vi "Log_subVI.vi"(6 "Data B":fxp<+,16,3>[](array[numeric]), 7 "Data A":fxp<+,16,3>[](array[numeric]), 8 "error in (no error)":errorcluster, 9 "Path":path, 10 "Samples to Read":dbl, 11 "Amplitude (V)":dbl) -> (0 "error out":errorcluster, 3 "Echo":dbl[][](graph))   [LabVIEW 2017]
doc: "Logs data from two separate channels and writes them to a single file on disk."
uses:
  <vilib>/Utility/file.llb/Write Delimited Spreadsheet (string).vi
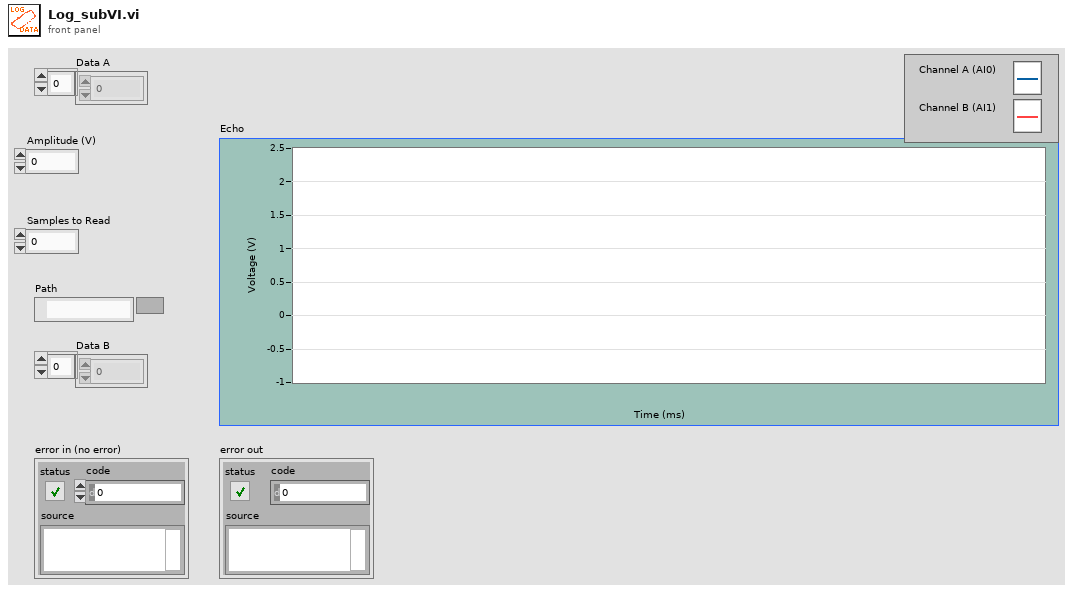
[diagram p1: front panel]
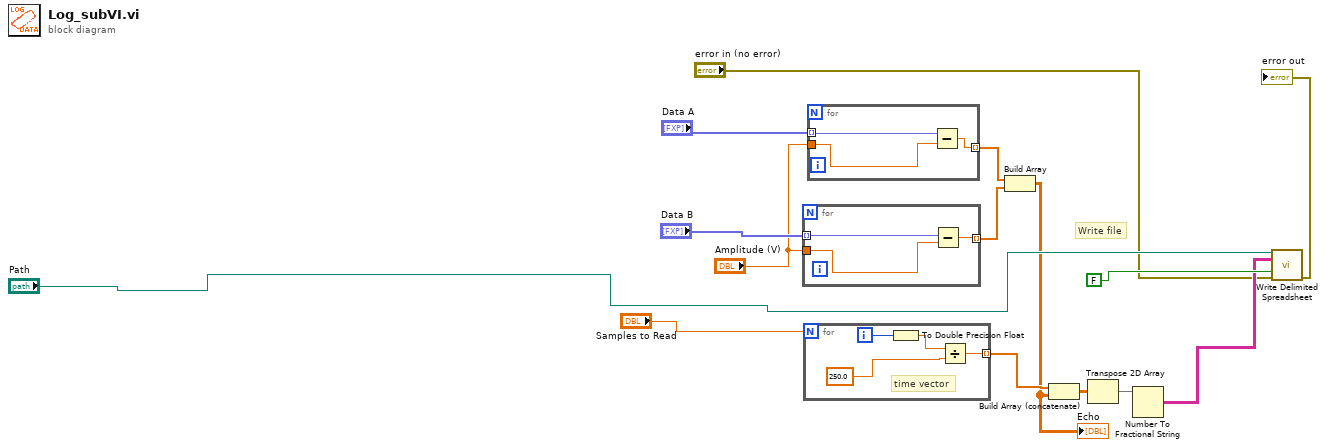
[diagram p0: block diagram]
diagram:
  # "Write file"
  n1 = for {
    tunnel: "Data B" -> [w18] mode=indexing
    tunnel: [w17] -> w12 mode=indexing
    tunnel: "Amplitude (V)" -> [w16]
    n2 = Subtract(x=w18, y=w16) -> (x-y=w17:dbl)
  }
  n3 = for {
    N: "Samples to Read" -> [_]
    tunnel: [w20] -> w10 mode=indexing
    i -> [w22]
    # "time vector"
    n4 = To Double Precision Float(number=w22) -> (double precision float=w21:dbl)
    n5 = Divide(x=w21, y=250.0) -> (x/y=w20:dbl)
  }
  n6 = for {
    tunnel: "Data A" -> [w25] mode=indexing
    tunnel: [w24] -> w11 mode=indexing
    tunnel: "Amplitude (V)" -> [w23]
    n7 = Subtract(x=w25, y=w23) -> (x-y=w24:dbl)
  }
  n8 = Build Array(w11, w12) -> (w7:dbl[][])
  "Echo" <- w7
  n9 = Build Array (concatenate)(w10, w7) -> (w8:dbl[][])
  n10 = Transpose 2D Array(2D array=w8) -> (transposed array=w9:dbl[][])
  n11 = Number To Fractional String(number=w9) -> (F-format string=w13:string[][])  [unwired: 3 in]
  n12 = call-poly <vilib>:"Write Delimited Spreadsheet.vi"("file path (dialog if empty)"="Path", "2D data"=w13, "append to file? (new file:F)"=FALSE, "error in (no error)"="error in (no error)") -> ("error out"=→"error out":errorcluster)  [unwired: 10 in, 1 out]
